vi "Event Timing Capture 1.0 In Place Output Read Structure.vi"(7 "Device outputs in":dbl[](array[numeric]), 8 "error in (no error)":errorcluster, 9 "FPGA ref in":T1, 11 "1.0.0 Event Timing Capture in":T2) -> (0 "error out":errorcluster, 1 "FPGA ref out":T1, 3 "1.0.0 Event Timing Capture out":T2, 5 "Device outputs out":dbl[](array[numeric]))   [LabVIEW 2020, in "Engine Simulation Toolkit Engine.lvlib"]
uses:
  Engine Simulation Toolkit Engine.lvlib
  Shared/1.0 Event Timing Capture Engine Data.ctl
  Shared/1.0 Event Timing Capture FIFO Idxs.ctl
  Event Timing Capture 1.0 Output Ref.ctl
  <vilib>/Utility/error.llb/Error Cluster From Error Code.vi
  <vilib>/rvi/errors/niLvFpgaAdjustHostInterfaceError.vi
  <vilib>/rvi/interface/nirviReadWriteControl/nirviReadWriteControl.xnode
  NiFpgaLv.dll
  <vilib>/rvi/interface/Simulation/niFpgaSimulationCallBeginRW.vi
  Shared/Engine Simulation Toolkit Shared.lvlib
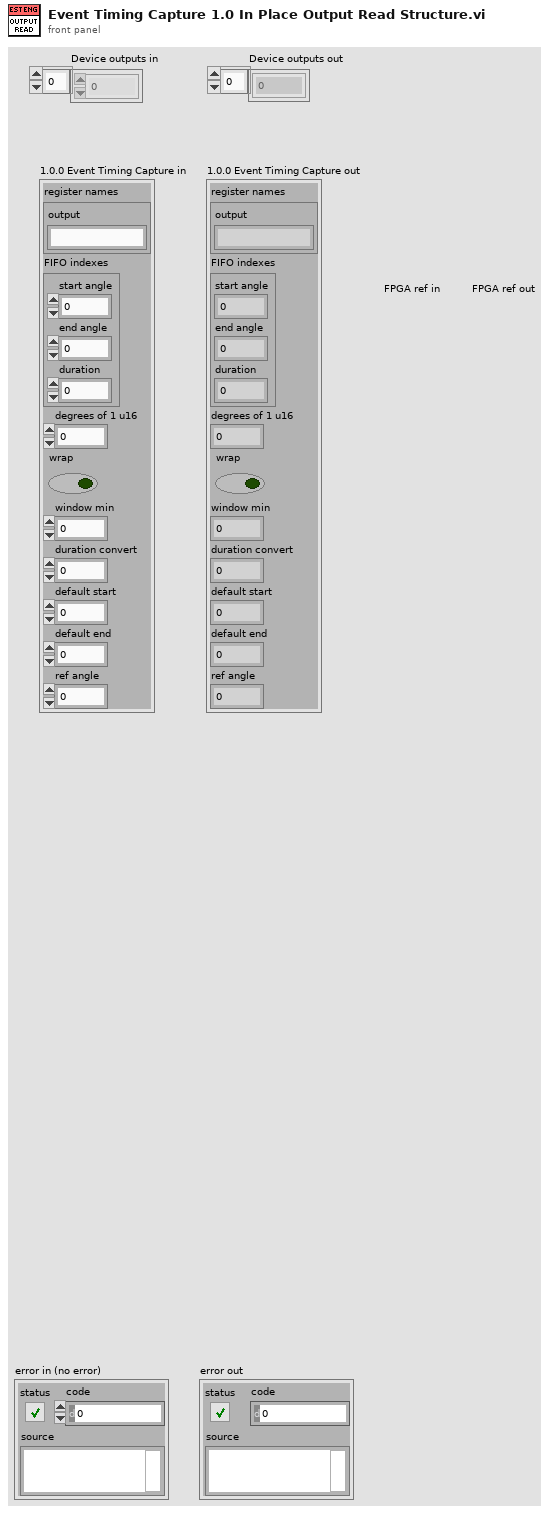
[diagram p1: front panel]
types:
  T1 = typedef "Engine Simulation Toolkit Engine.lvlib/Event Timing Capture 1.0 Output Ref.ctl" = refnum<k20>
  T2 = typedef "Engine Simulation Toolkit Shared.lvlib/1.0 Event Timing Capture Engine Data.ctl" = cluster{"register names":cluster{"output":string}, "FIFO indexes":T3, "degrees of 1 u16":dbl, "wrap":bool, "window min":u16, "duration convert":dbl, "default start":dbl, "default end":dbl, "ref angle":dbl}
  T3 = typedef "Engine Simulation Toolkit Shared.lvlib/1.0 Event Timing Capture FIFO Idxs.ctl" = cluster{"start angle":i32, "end angle":i32, "duration":i32}
  T4 = cluster{"Start":u16, "End":u16, "Duration (tics)":fxp<+,18,18>, "Event present":bool}
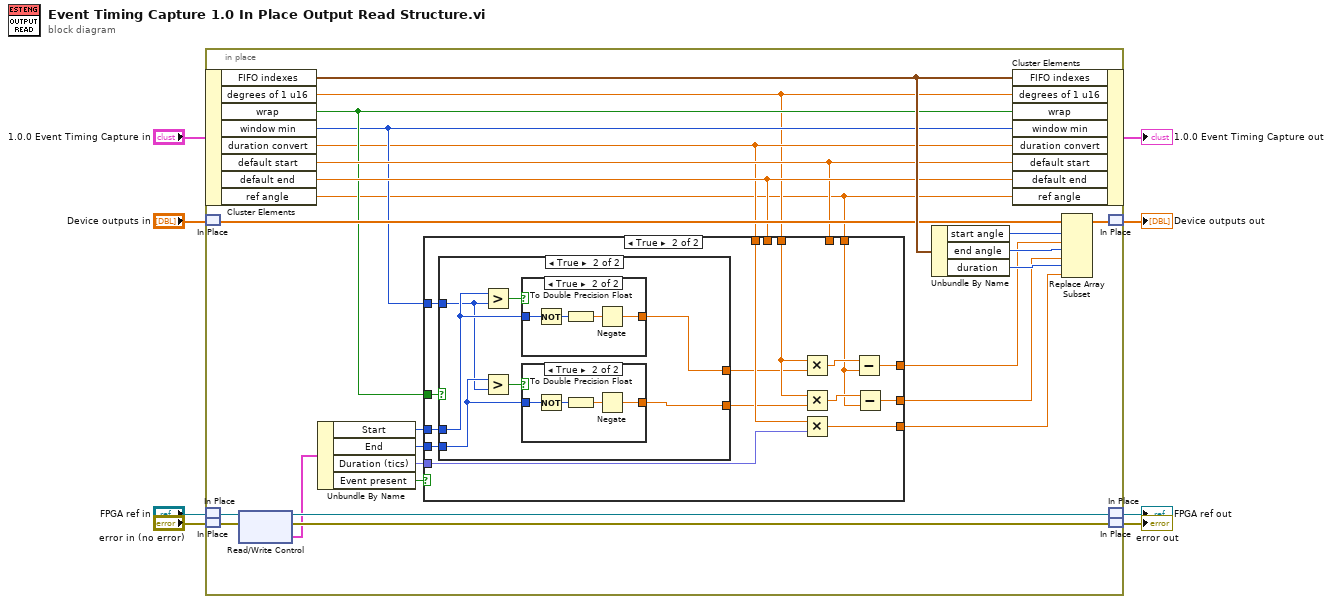
[diagram p0: block diagram]
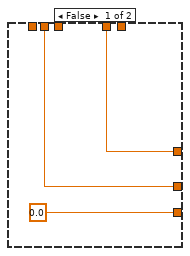
[diagram p2: hidden frame]
diagram:
  n1 = in-place {
    n2 = in-place-cluster #1("1.0.0 Event Timing Capture in") -> ("FIFO indexes"=w27:T3, "degrees of 1 u16"=w10:dbl, "wrap"=w13:bool, "window min"=w12:u16, "duration convert"=w11:dbl, "default start"=w18:dbl, "default end"=w20:dbl, "ref angle"=w9:dbl)
    n3 = in-place-match #2("Device outputs in") -> (w23:dbl[])
    n4 = in-place-match #3("FPGA ref in") -> (w32:T1)
    n5 = in-place-match #4("error in (no error)") -> (w33:errorcluster)
    n6 = xnode "Read/Write Control"("FPGA VI Reference In"=w32, "error in"=w33) -> ("FPGA VI Reference Out"=w31:T1, "error out"=w30:errorcluster, "Value"=w29:T4)
    n7 = Unbundle By Name(w29) -> ("Start"=w14:u16, "End"=w15:u16, "Duration (tics)"=w16:fxp<+,18,18>, "Event present"=w28:bool)
    n8 = case shown="True" w28 {
      tunnel: [0.0 ("new element/subarray") w45] -> w21
      tunnel: w20 -> [w34 _]
      tunnel: [w34 w38] -> w19
      tunnel: w18 -> [w35 _]
      tunnel: [w35 w39] -> w17
      tunnel: w16 -> [_ w44]
      tunnel: w15 -> [_ w49]
      tunnel: w14 -> [_ w50]
      tunnel: w13 -> [_ w51]
      tunnel: w12 -> [_ w48]
      tunnel: w11 -> [_ w43]
      tunnel: w10 -> [_ w42]
      tunnel: w9 -> [_ w37]
      frame False {
      }
      frame True {
        n9 = case shown="True" w51 {
          tunnel: w50 -> [w53 w59]
          tunnel: w49 -> [w52 w56]
          tunnel: w48 -> [_ w55]
          tunnel: [w53 w58] -> w41
          tunnel: [w52 w54] -> w40
          frame False {
          }
          frame True {
            n10 = Greater?(x=w59, y=w55) -> (0:w60:bool)
            n11 = Greater?(x=w56, y=w55) -> (0:w57:bool)
            n12 = case shown="True" w60 {
              tunnel: w59 -> [w66 w68]
              tunnel: [w66 w67] -> w58
              frame False {
              }
              frame True {
                n13 = Not(x=w68) -> (.not. x?=w69:u16)
                n14 = To Double Precision Float(number=w69) -> (double precision float=w70:dbl)
                n15 = Negate(x=w70) -> (-x=w67:dbl)
              }
            }
            n16 = case shown="True" w57 {
              tunnel: w56 -> [w61 w63]
              tunnel: [w61 w62] -> w54
              frame False {
              }
              frame True {
                n17 = Not(x=w63) -> (.not. x?=w64:u16)
                n18 = To Double Precision Float(number=w64) -> (double precision float=w65:dbl)
                n19 = Negate(x=w65) -> (-x=w62:dbl)
              }
            }
          }
        }
        n20 = Multiply(x=w42, y=w41) -> (x*y=w47:dbl)
        n21 = Multiply(x=w42, y=w40) -> (x*y=w46:dbl)
        n22 = Multiply(x=w43, y=w44) -> (x*y=w45:dbl)
        n23 = Subtract(x=w47, y=w37) -> (x-y=w39:dbl)
        n24 = Subtract(x=w46, y=w37) -> (x-y=w38:dbl)
      }
    }
    n25 = Unbundle By Name(w27) -> ("start angle"=w24:i32, "end angle"=w25:i32, "duration"=w26:i32)
    n26 = in-place-cluster #1("FIFO indexes"=w27, "degrees of 1 u16"=w10, "wrap"=w13, "window min"=w12, "duration convert"=w11, "default start"=w18, "default end"=w20, "ref angle"=w9) -> (→"1.0.0 Event Timing Capture out":T2)
    n27 = Replace Array Subset(array=w23, new element #1=w17, index #1=w24, new element #2=w19, index #2=w25, new element #3=w21, index #3=w26) -> (w22:dbl[])
    n28 = in-place-match #2(w22) -> (→"Device outputs out":dbl[])
    n29 = in-place-match #3(w31) -> (→"FPGA ref out":T1)
    n30 = in-place-match #4(w30) -> (→"error out":errorcluster)
  }
